vi "loadPositions.vi"() -> (0 "positions":cluster{string, string}[](array[cluster]))   [LabVIEW 2013]
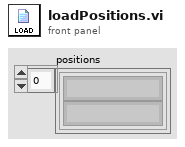
[diagram p1: front panel]
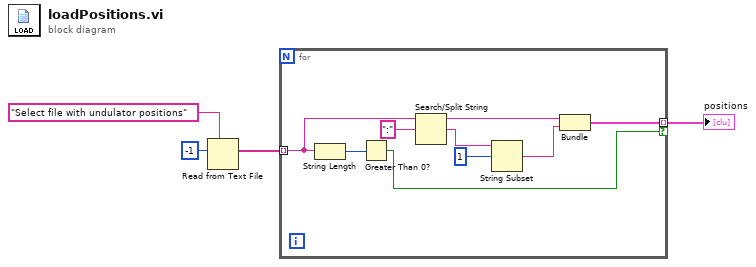
[diagram p0: block diagram]
diagram:
  n1 = Read from Text File(prompt (Open existing file)="Select file with undulator positions", count=-1) -> (text=w4:string[])  [unwired: 2 in, 3 out]
  n2 = for {
    tunnel: w4 -> [w12] mode=indexing
    tunnel: [w6] -> w2 mode=indexing if=w5
    n3 = String Length(string=w12) -> (length=w13:i32)
    n4 = Greater Than 0?(x=w13) -> (x > 0?=w5:bool)
    n5 = Search/Split String(string=w12, search string/char (-)=":") -> (substring before match=w8:string, match + rest of string=w10:string)  [unwired: 1 in, 1 out]
    n6 = String Subset(string=w10, offset (0)=1 ("offset")) -> (substring=w7:string)  [unwired: 1 in]
    n7 = Bundle(w8, w7) -> (w6:cluster{string, string})  [unwired: 1 in]
  }
  "positions" <- w2
